vi "Angulo_Declinacion.vi"(1 "n":dbl) -> (0 "Declinación":dbl(knob) scale=-23.45..23.45)   [LabVIEW 2020]
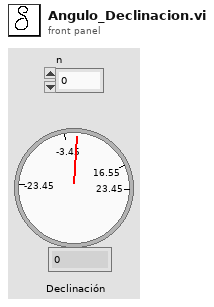
[diagram p1: front panel]
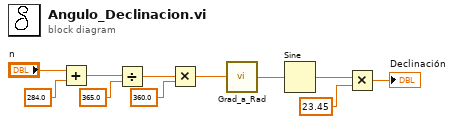
[diagram p0: block diagram]
diagram:
  n1 = Add(x="n", y=284.0) -> (x+y=w10:dbl)
  n2 = Divide(x=w10, y=365.0) -> (x/y=w9:dbl)
  n3 = Multiply(x=w9, y=360.0) -> (x*y=w5:dbl)
  n4 = call "Grad_a_Rad.vi"("Grados"=w5) -> ("Radianes"=w4:dbl)
  n5 = Sine(x=w4) -> (sin(x)=w3:dbl)
  n6 = Multiply(x=w3, y=23.45) -> (x*y=→"Declinación":dbl)
